vi "Read TOML File (LV).vi"(7 "Default Value":variant, 8 "error in (no error)":errorcluster, 11 "file path (use dialog)":path) -> (0 "error out":errorcluster, 3 "Value":variant)   [LabVIEW 2015, in "TOML.lvlib"]
uses:
  TOML.lvlib
  TOML Value.ctl
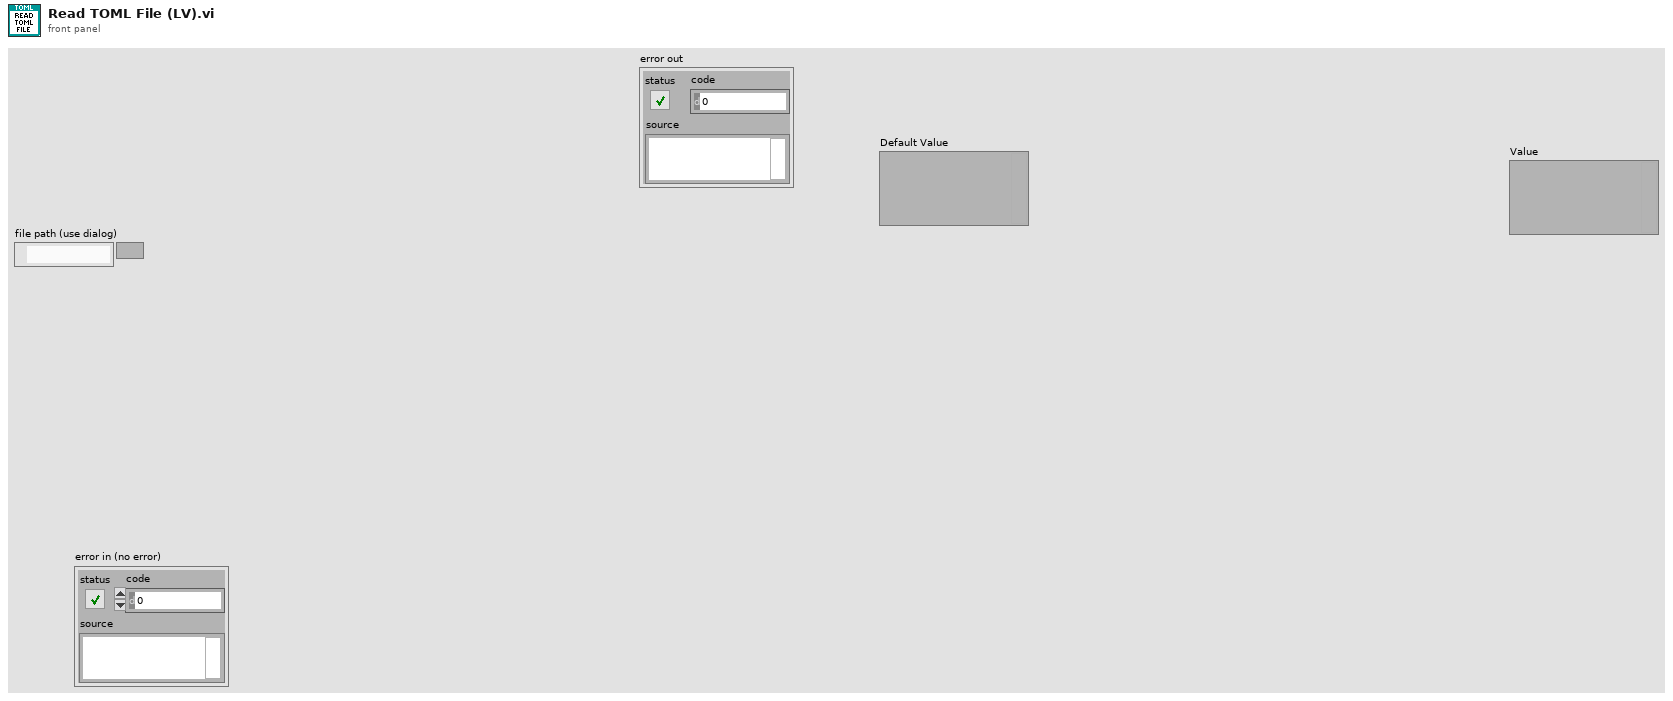
[diagram p1: front panel]
types:
  T1 = enum16{"Table", "Array", "String", "Integer", "Float", "Boolean", "Offset Date-Time", "Local Date-Time", "Local Date", "Local Time"}
  T2 = typedef "TOML.lvlib/TOML Value.ctl" = cluster{"\\type":enum16{"Table", "Array", "String", "Integer", "Float", "Boolean", "Offset Date-Time", "Local Date-Time", "Local Date", "Local Time"}, "ÿýÿýÿýÿýÿýÿþÿýÿýÿý\"TOML.lvlib:TOML Key-Value Pair.ctlÿýÿýÿýÿýÿýÿþÿýÿýÿýTOML.lvlib:TOML Value.ctl$$":variant}
  T3 = enum16{"open", "replace", "create", "open or create", "replace or create", "replace or create with confirmation"}
  T4 = typedef "TOML.lvlib/TOML Key-Value Pair.ctl" = cluster{"Key":string, "Value":T2}
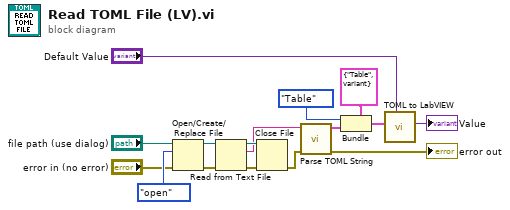
[diagram p0: block diagram]
diagram:
  n1 = Open/Create/Replace File(file path (use dialog)="file path (use dialog)", error in="error in (no error)", operation (0:open)=T3."open") -> (refnum out=w13:refnum<file>, error out=w14:errorcluster)  [unwired: 3 in, 1 out]
  n2 = Read from Text File(file (use dialog)=w13, error in=w14) -> (refnum out=w11:refnum<file>, text=w9:string, error out=w12:errorcluster)  [unwired: 2 in, 1 out]
  n3 = Close File(refnum=w11, error in=w12) -> (error out=w8:errorcluster)  [unwired: 1 out]
  n4 = call "Parse TOML String.vi"("error in (no error)"=w8, "String"=w9) -> ("error out"=→"error out":errorcluster, "Table"=w5:T4[])  [unwired: 8 in]
  n5 = Bundle(cluster=T2 {"\\type"=enum."Table", "ÿýÿýÿýÿýÿýÿþÿýÿýÿý\"TOML.lvlib:TOML Key-Value Pair.ctlÿýÿýÿýÿýÿýÿþÿýÿýÿýTOML.lvlib:TOML Value.ctl$$"=variant} ("Value"), "\\type"=T1."Table" ("Type"), "ÿýÿýÿýÿýÿýÿþÿýÿýÿý\"TOML.lvlib:TOML Key-Value Pair.ctlÿýÿýÿýÿýÿýÿþÿýÿýÿýTOML.lvlib:TOML Value.ctl$$"=w5) -> (w4:T2)
  n6 = call "TOML to LabVIEW.vi"("Default Value"="Default Value", "TOML Value"=w4) -> ("LV Value"=→"Value":variant)  [unwired: 9 in]
